vi "题目六.vi"() -> ()   [LabVIEW 2017]
panel:
  out "字符串":string
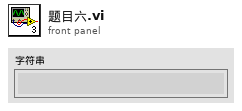
[diagram p1: front panel]
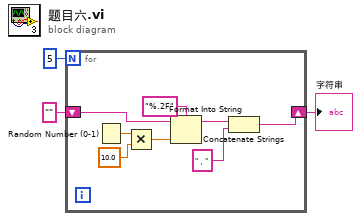
[diagram p0: block diagram]
diagram:
  n1 = for {
    N: 5 -> [_]
    shift-right: [w4] -> w1
    shift-left: "" -> [w5]
    n2 = Random Number (0-1)() -> (number: 0 to 1=w11:dbl)
    n3 = Multiply(x=w11, y=10.0) -> (x*y=w9:dbl)
    n4 = Format Into String(format string="%.2F" ("格式字符串"), initial string=w5, w9) -> (resulting string=w7:string)  [unwired: 1 in, 1 out]
    n5 = Concatenate Strings(w7, "，" ("字符串")) -> (w4:string)
  }
  "字符串" <- w1
